vi "Filter.vi"(10 "Fs":dbl, 11 "Input":dbl) -> (3 "Filtered signal":dbl)   [LabVIEW 2016]
doc: "Highpass Lowpass and Bandstop filter"
uses:
  <vilib>/Analysis/3filter.llb/Filter Passband Type.ctl
  <vilib>/ptbypt/NI_PtbyPt.lvlib
  <vilib>/Analysis/NI_AALBase.lvlib
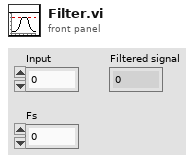
[diagram p1: front panel]
types:
  T1 = typedef "NI_AALBase.lvlib/Filter Passband Type.ctl" = enum32{"Lowpass", "Highpass", "Bandpass", "Bandstop"}
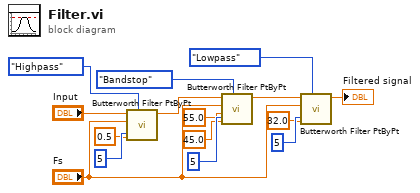
[diagram p0: block diagram]
diagram:
  n1 = call <vilib>:"Butterworth Filter PtByPt.vi"("order"=5, "filter type"=Filter_Passband_Type."Highpass", "low cutoff freq: fl"=0.5, "sampling freq: fs"="Fs", "x"="Input") -> ("Filtered x"=w4:dbl)  [unwired: 4 in, 1 out]
  n2 = call <vilib>:"Butterworth Filter PtByPt.vi"("order"=5, "filter type"=Filter_Passband_Type."Bandstop", "low cutoff freq: fl"=45.0, "high cutoff freq: fh"=55.0, "sampling freq: fs"="Fs", "x"=w4) -> ("Filtered x"=w9:dbl)  [unwired: 3 in, 1 out]
  n3 = call <vilib>:"Butterworth Filter PtByPt.vi"("order"=5, "filter type"=Filter_Passband_Type."Lowpass", "low cutoff freq: fl"=32.0, "sampling freq: fs"="Fs", "x"=w9) -> ("Filtered x"=→"Filtered signal":dbl)  [unwired: 4 in, 1 out]
